vi "test no change passes.vi"(8 "error in (no error)":errorcluster, 11 "TestCase in":refnum<class "Testing Approval Tests.lvclass">) -> (0 "error out":errorcluster, 3 "TestCase out":refnum<class "Testing Approval Tests.lvclass">)   [LabVIEW 2020, in "Testing Approval Tests.lvclass"]
uses:
  Testing Approval Tests.lvclass
  <vilib>/addons/_JKI Toolkits/VI Tester/TestCase.llb/TestCase.lvclass
  Approval Tests/Approval Tests.lvlib
  C:/Program Files/National Instruments/LabVIEW 2020/vi.lib/addons/_JKI Toolkits/VI Tester/TestCase.llb/TestCase.lvclass
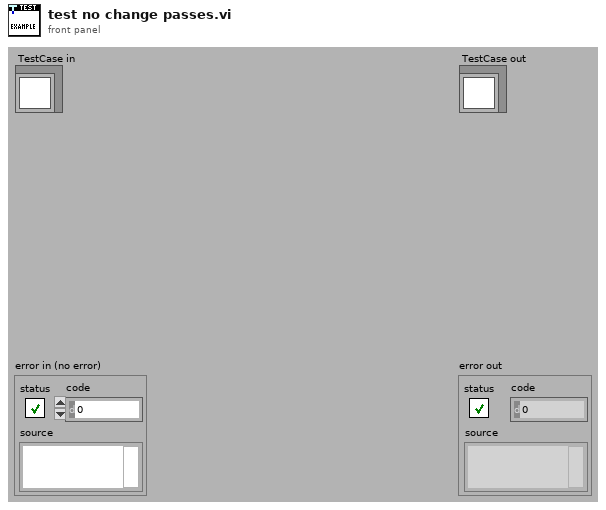
[diagram p1: front panel]
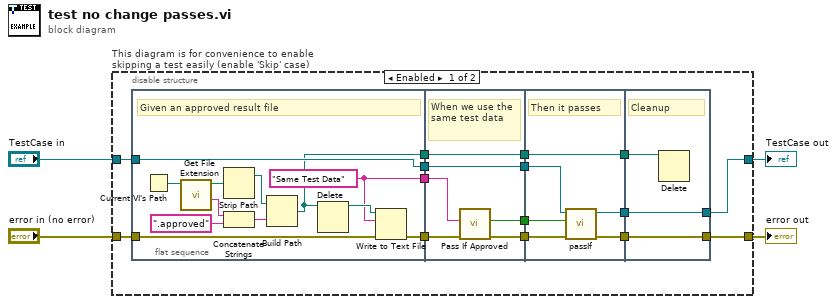
[diagram p0: block diagram]
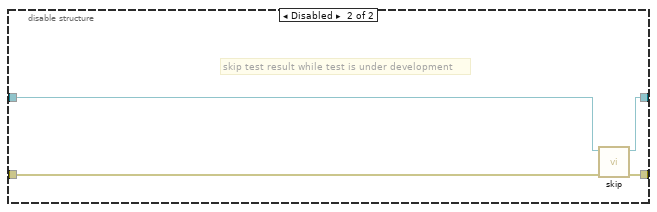
[diagram p2: hidden frame]
diagram:
  n1 = disable-structure "This diagram is for convenience to enable skipping a test easily (enable 'Skip' case)" shown="Enabled" {
    disable-tunnel: "TestCase in" -> [w11 w50]
    disable-tunnel: [w10 w48] -> w1
    disable-tunnel: [w18 w49] -> w3
    disable-tunnel: "error in (no error)" -> [w19 w47]
    frame Enabled {
      n2 = flat-sequence {
        tunnel: w19 -> [w24]
        tunnel: [w23] -> w17
        tunnel: [w31] -> w12
        tunnel: w11 -> [w31]
        tunnel: [w21] -> w9
        tunnel: [w20] -> w5
        tunnel: w17 -> [w36]
        tunnel: [w35] -> w16
        tunnel: [w37] -> w13
        tunnel: w12 -> [w37]
        tunnel: w9 -> [w33]
        tunnel: [w32] -> w8
        tunnel: [w34] -> w6
        tunnel: w5 -> [w34]
        tunnel: w16 -> [w43]
        tunnel: [w42] -> w15
        tunnel: [w40] -> w14
        tunnel: w13 -> [w41]
        tunnel: w8 -> [w39]
        tunnel: [w38] -> w7
        tunnel: w6 -> [w38]
        tunnel: [w46] -> w18
        tunnel: w15 -> [w46]
        tunnel: [w45] -> w10
        tunnel: w14 -> [w45]
        tunnel: w7 -> [w44]
        frame #0 {
          w21 = "Same Test Data"
          # "Given an approved result file"
          n3 = Current VI's Path() -> (path=w30:path)
          n4 = call <vilib>:"Get File Extension.vi"("file"=w30) -> ("filename without extension"=w27:string, "dup file"=w29:path)  [unwired: 6 in, 3 out]
          n5 = Strip Path(path=w29) -> (stripped path=w28:path)  [unwired: 1 out]
          n6 = Concatenate Strings(w27, ".approved" ("string")) -> (w26:string)
          n7 = Build Path(base path=w28, name or relative path=w26) -> (appended path=w20:path)
          n8 = Delete(path (use dialog)=w20) -> (deleted path=w22:path)  [unwired: 4 in, 2 out]
          n9 = Write to Text File(file (use dialog)=w22, text=w21, error in=w24) -> (error out=w23:errorcluster)  [unwired: 1 in, 2 out]
        }
        frame #1 {
          # "When we use the same test data"
          n10 = call "Pass If Approved.vi"("error in"=w36, "Test Data"=w33) -> ("error out"=w35:errorcluster, "Passed?"=w32:bool)  [unwired: 7 in, 1 out]
        }
        frame #2 {
          # "Then it passes"
          n11 = call-dynamic "passIf.vi"("error in (no error)"=w43, "pass"=w39, "TestCase in"=w41) -> ("error out"=w42:errorcluster, "TestCase out"=w40:refnum<class "Testing Approval Tests.lvclass">)  [unwired: 7 in]
        }
        frame #3 {
          # "Cleanup"
          n12 = Delete(path (use dialog)=w44) -> ()  [unwired: 4 in, 3 out]
        }
      }
    }
    frame Disabled {
      # "skip test result while test is under development"
      n13 = call <vilib>:"skip.vi"("error in (no error)"=w47, "TestCase in"=w50) -> ("error out"=w49:errorcluster, "TestCase out"=w48:refnum<class "Testing Approval Tests.lvclass">)  [unwired: 8 in]
    }
  }
  "error out" <- w3
  "TestCase out" <- w1
